vi "Check File Path.vi"(8 "error in":errorcluster, 11 "Path to Check":path) -> (0 "error out":errorcluster, 1 "Path Modified?":bool, 2 "Original Path":path, 3 "Valid Path":path, 5 "File Changed?":string="Original path: ")   [LabVIEW 2024]
panel:
  in  "File Extension":string=".txt"
  # "Inputs"
  # "Outputs"
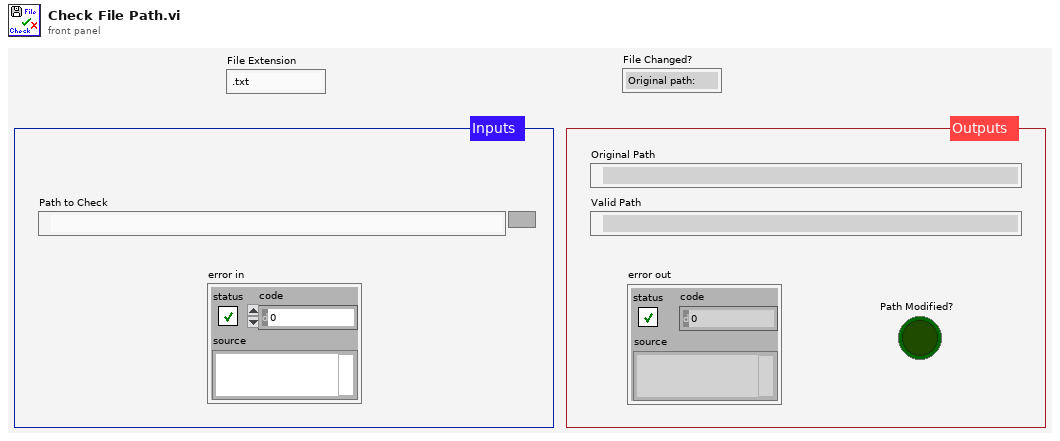
[diagram p1: front panel]
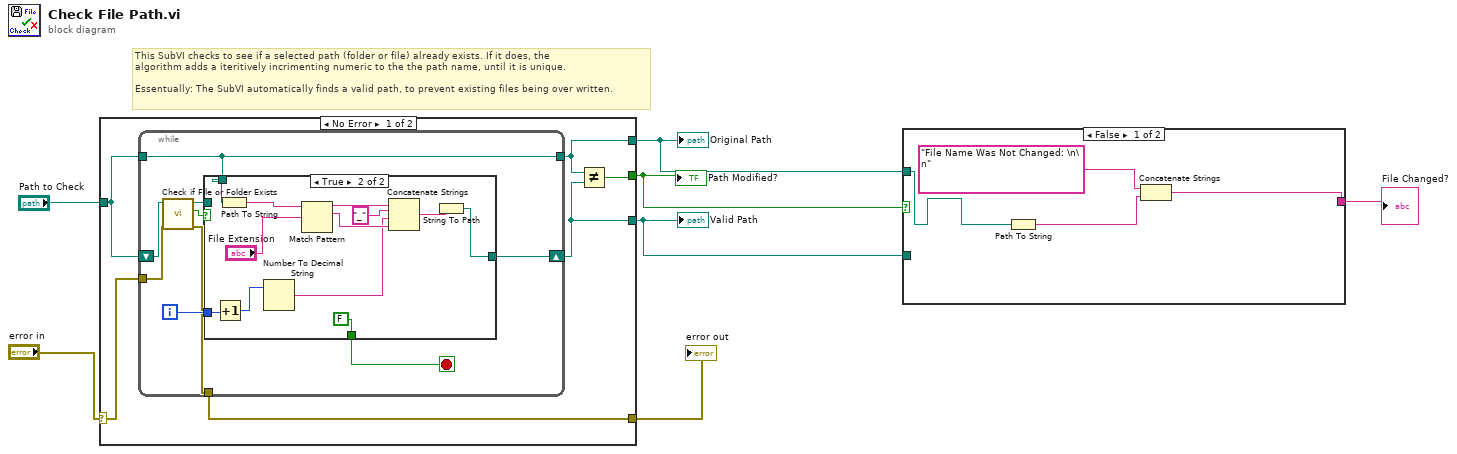
[diagram p0: block diagram]
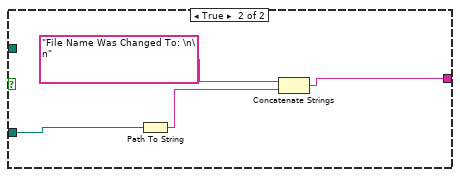
[diagram p2: hidden frame]
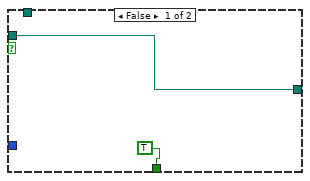
[diagram p3: hidden frame]
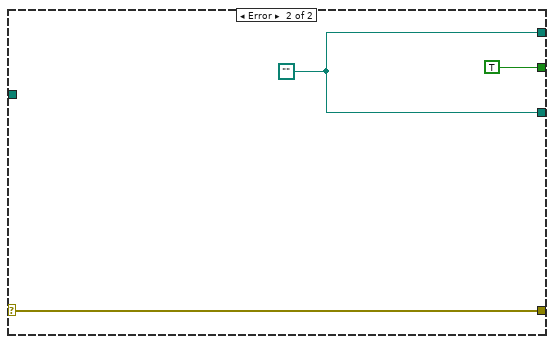
[diagram p4: hidden frame]
diagram:
  # "This SubVI checks to see if a selected path (folder or file) already exists. If it does, the \nalgorithm adds a iteritively incrimenting numeric to the the path name, until it is unique.\n\nEssentually: The SubVI automatically finds a valid path, to prevent existing files being over written."
  n1 = case shown="No Error" "error in" {
    selector: "error in" -> [w9 w38]
    tunnel: "Path to Check" -> [w10 _]
    tunnel: [w13 w37] -> w1
    tunnel: [w12 w37] -> w3
    tunnel: [w11 TRUE] -> w4
    tunnel: [w8 w38] -> w5
    frame No Error {
      n2 = while {
        shift-right: [w20] -> w12
        shift-left: w10 -> [w19]
        tunnel: [w16] -> w13
        tunnel: w10 -> [w16]
        tunnel: w9 -> [w15]
        tunnel: [w14] -> w8
        i -> [w18]
        stop <- w21 stop-if-true
        n3 = call <vilib>:"Check if File or Folder Exists.vi"("error in (no error)"=w15, "path"=w19) -> ("error out"=w14:errorcluster, "file or folder exists?"=w22:bool, "dup path"=w17:path)  [unwired: 7 in]
        n4 = case shown="True" w22 {
          tunnel: [TRUE FALSE] -> w21
          tunnel: w18 -> [_ w36]
          tunnel: [w23 w34] -> w20
          tunnel: w17 -> [w23 _]
          tunnel: w16 -> [_ w28]
          frame False {
          }
          frame True {
            n5 = Increment(x=w36) -> (x+1=w32:i32)
            n6 = Path To String(path=w28) -> (string=w31:string)
            n7 = Number To Decimal String(number=w32) -> (decimal integer string=w26:string)  [unwired: 1 in]
            n8 = Match Pattern(string=w31, regular expression="File Extension") -> (before substring=w29:string, match substring=w27:string)  [unwired: 1 in, 2 out]
            n9 = Concatenate Strings(w29, "_" ("string"), w26, w27) -> (w35:string)
            n10 = String To Path(string=w35) -> (path=w34:path)
          }
        }
      }
      n11 = Not Equal?(x=w13, y=w12) -> (x != y?=w11:bool)
    }
    frame Error {
      w37 = path ""
    }
  }
  "Valid Path" <- w3
  "Path Modified?" <- w4
  "Original Path" <- w1
  "error out" <- w5
  n12 = case shown="False" w4 {
    tunnel: w3 -> [_ w44]
    tunnel: [w41 w47] -> w2
    tunnel: w1 -> [w40 _]
    frame False {
      n13 = Path To String(path=w40) -> (string=w42:string)
      n14 = Concatenate Strings("File Name Was Not Changed: \n\n" ("File Changed? 2"), w42) -> (w41:string)
    }
    frame True {
      n15 = Path To String(path=w44) -> (string=w45:string)
      n16 = Concatenate Strings("File Name Was Changed To: \n\n" ("File Extension 2"), w45) -> (w47:string)
    }
  }
  "File Changed?" <- w2
